vi "test Detect Changed Indices.vi"(8 "error in (no error)":errorcluster, 11 "TestCase in":refnum<class "Shared VIs.lvclass">) -> (0 "error out":errorcluster, 3 "TestCase out":refnum<class "Shared VIs.lvclass">)   [LabVIEW 2024, in "Shared VIs.lvclass"]
uses:
  Shared VIs.lvclass
  c8128e39-ba4a-4d39-8bf0-919f2f8f5ee1.vi
  f757781e-0541-4624-9f36-0c3754dd0849.vi
  <vilib>/addons/_JKI Toolkits/VI Tester/TestCase.llb/TestCase.lvclass
  C:/Program Files/National Instruments/LabVIEW 2024/vi.lib/addons/_JKI Toolkits/VI Tester/TestCase.llb/TestCase.lvclass
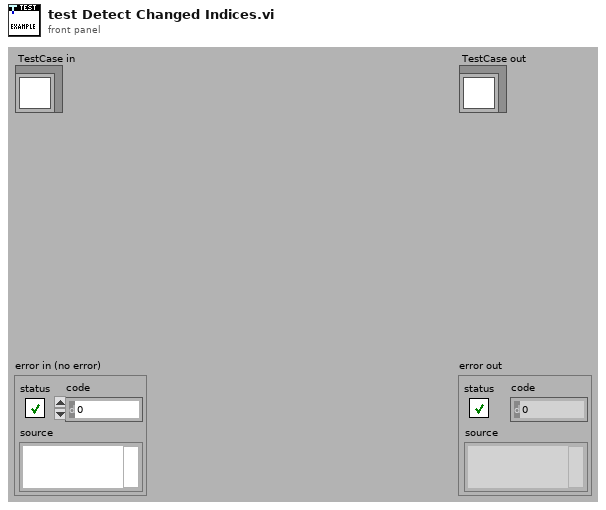
[diagram p1: front panel]
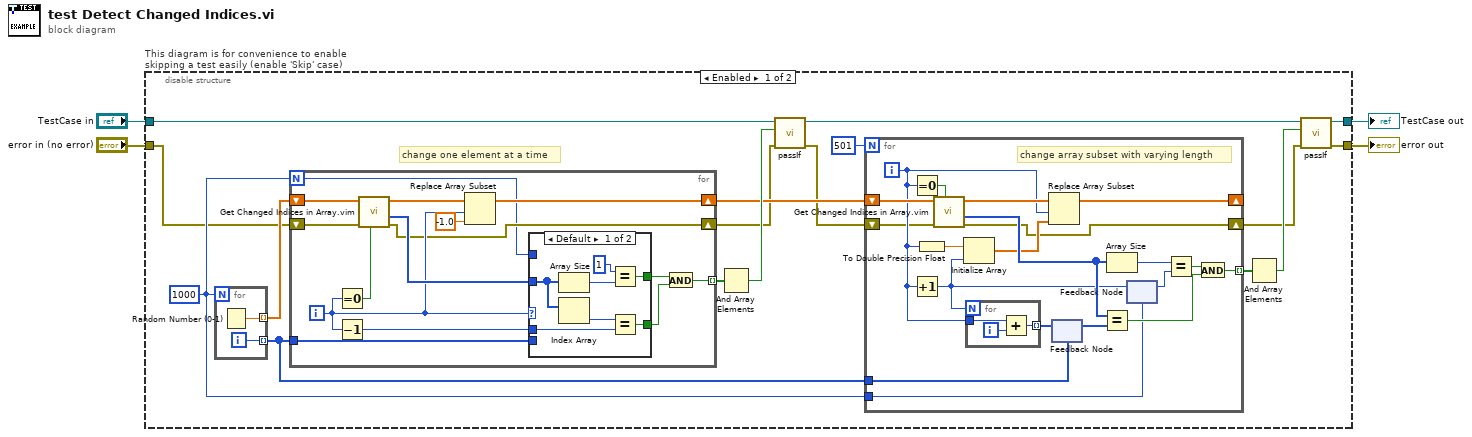
[diagram p0: block diagram]
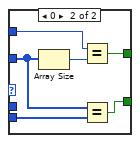
[diagram p2: hidden frame]
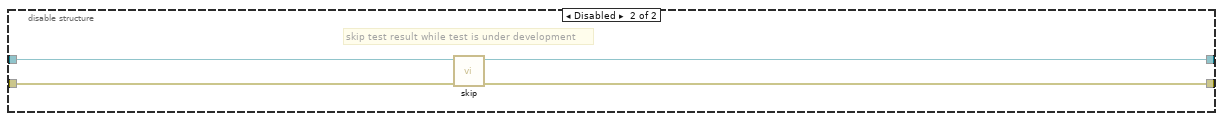
[diagram p3: hidden frame]
diagram:
  n1 = disable-structure "This diagram is for convenience to enable skipping a test easily (enable 'Skip' case)" shown="Enabled" {
    disable-tunnel: "TestCase in" -> [w21 w78]
    disable-tunnel: [w9 w76] -> w1
    disable-tunnel: [w10 w77] -> w3
    disable-tunnel: "error in (no error)" -> [w7 w75]
    frame Enabled {
      w15 = 1000
      # "change one element at a time"
      n2 = for {
        N: w15 -> [_]
        tunnel: [w74] -> w20 mode=indexing
        tunnel: [w73] -> w16 mode=indexing
        i -> [w73]
        n3 = Random Number (0-1)() -> (number: 0 to 1=w74:dbl)
      }
      n4 = for {
        N: w15 -> [w45]
        shift-right: [w56] -> w17
        shift-left: w20 -> [w59]
        tunnel: w16 -> [w53]
        tunnel: [w50] -> w19 mode=indexing
        shift-right: [w46] -> w8
        shift-left: w7 -> [w47]
        i -> [w48]
        n5 = Equal To 0?(x=w48) -> (x = 0?=w58:bool)
        n6 = Decrement(x=w48) -> (x-1=w49:i32)
        n7 = call "Get Changed Indices in Array.vim"("reset"=w58, "error in"=w47, "data in"=w59) -> ("error out"=w46:errorcluster, "changed indices"=w54:i32[], "data out"=w57:dbl[])  [unwired: 4 in]
        n8 = Replace Array Subset(array=w57, new element=-1.0 ("new element/subarray"), index=w48) -> (w56:dbl[])
        n9 = case shown="Default" w48 {
          tunnel: w54 -> [w64 w70]
          tunnel: w45 -> [_ w71]
          tunnel: w53 -> [_ w69]
          tunnel: [w61 w68] -> w52
          tunnel: [w60 w67] -> w51
          tunnel: w49 -> [w65 _]
          frame Default {
            n10 = Array Size(array=w64) -> (size(s)=w63:i32)
            n11 = Index Array(array=w64) -> (element=w66:i32)  [unwired: 1 in]
            n12 = Equal?(x=1 ("y"), y=w63) -> (x = y?=w60:bool)
            n13 = Equal?(x=w66, y=w65) -> (x = y?=w61:bool)
          }
          frame 0 {
            n14 = Array Size(array=w70) -> (size(s)=w72:i32)
            n15 = Equal?(x=w71, y=w72) -> (x = y?=w67:bool)
            n16 = Equal?(x=w70, y=w69) -> (x = y?=w68:bool)
          }
        }
        n17 = And(x=w51, y=w52) -> (x .and. y?=w50:bool)
      }
      n18 = And Array Elements(Boolean array=w19) -> (logical AND=w18:bool)
      n19 = call-dynamic "passIf.vi"("error in (no error)"=w8, "pass"=w18, "TestCase in"=w21) -> ("error out"=w6:errorcluster, "TestCase out"=w11:refnum<class "Shared VIs.lvclass">)  [unwired: 7 in]
      n20 = for {
        N: 501 -> [_]
        shift-right: [w38] -> _
        shift-left: w17 -> [w41]
        tunnel: w15 -> [w26]
        tunnel: [w34] -> w12 mode=indexing
        tunnel: w16 -> [w27]
        shift-right: [w22] -> w5
        shift-left: w6 -> [w23]
        i -> [w30]
        # "change array subset with varying length"
        n21 = Equal To 0?(x=w30) -> (x = 0?=w40:bool)
        n22 = Increment(x=w30) -> (x+1=w25:i32)
        n23 = To Double Precision Float(number=w30) -> (double precision float=w31:dbl)
        n24 = call "Get Changed Indices in Array.vim"("reset"=w40, "error in"=w23, "data in"=w41) -> ("error out"=w22:errorcluster, "changed indices"=w37:i32[], "data out"=w39:dbl[])  [unwired: 4 in]
        n25 = Initialize Array(w31, w25) -> (w33:dbl[])
        n26 = for {
          N: w25 -> [_]
          tunnel: w30 -> [w43]
          tunnel: [w42] -> w29 mode=indexing
          i -> [w44]
          n27 = Add(x=w43, y=w44) -> (x+y=w42:i32)
        }
        n28 = Replace Array Subset(array=w39, new element=w33, index=w30) -> (w38:dbl[])
        n29 = feedback #1(w27) -> (w28:i32[])
        n30 = feedback-in #1(w29) -> ()
        n31 = Equal?(x=w37, y=w28) -> (x = y?=w36:bool)
        n32 = Array Size(array=w37) -> (size(s)=w24:i32)
        n33 = feedback-in #2(w25) -> ()
        n34 = feedback #2(w26) -> (w32:i32)
        n35 = Equal?(x=w24, y=w32) -> (x = y?=w35:bool)
        n36 = And(x=w35, y=w36) -> (x .and. y?=w34:bool)
      }
      n37 = And Array Elements(Boolean array=w12) -> (logical AND=w13:bool)
      n38 = call-dynamic "passIf.vi"("error in (no error)"=w5, "pass"=w13, "TestCase in"=w11) -> ("error out"=w10:errorcluster, "TestCase out"=w9:refnum<class "Shared VIs.lvclass">)  [unwired: 7 in]
    }
    frame Disabled {
      # "skip test result while test is under development"
      n39 = call <vilib>:"skip.vi"("error in (no error)"=w75, "TestCase in"=w78) -> ("error out"=w77:errorcluster, "TestCase out"=w76:refnum<class "Shared VIs.lvclass">)  [unwired: 8 in]
    }
  }
  "error out" <- w3
  "TestCase out" <- w1
